vi "Destroy Broadcast Events.vi"(8 "error in (no error)":errorcluster) -> (0 "error out":errorcluster)   [LabVIEW 2015, in "Thermal Chamber Controller_DQMH.lvlib"]
doc: "Destroy the broadcast events, even if there is an incoming error.\n\n<b>NOTE</b>: The contents of this VI are automatically generated and modified by the <b>Tools > Delacor > DQMH</b> utilities. Consider using those utilities instead of making your own modifications to this VI.\n_____\nBased on Delacor QMH Project Template 2.0.0.62.\n____\nDelacor QMH Thermal Chamber Examples 4.0.0.21\nCopyright (c) 2018, Delacor"
uses:
  Thermal Chamber Controller_DQMH.lvlib
panel:
  # "NOTE: The contents of this VI are automatically generated and modified by the Tools > Delacor > DQMH utilities. Consider using those utilities instead of making your own modifications to this VI."
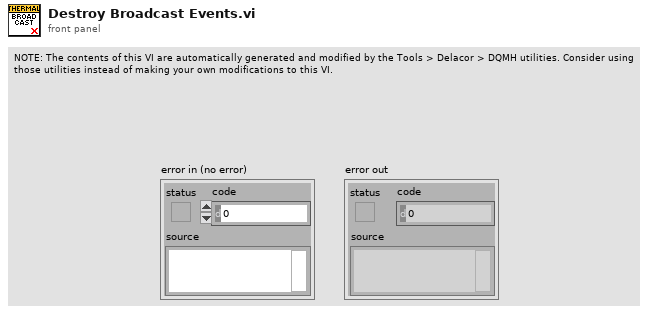
[diagram p1: front panel]
types:
  T1 = typedef "Thermal Chamber Controller_DQMH.lvlib/Broadcast Events--cluster.ctl" = cluster{"Module Did Init":refnum<user-event>, "Status Updated":refnum<user-event>, "Error Reported":refnum<user-event>, "Module Did Stop":refnum<user-event>, "Update Module Execution Status":refnum<user-event>, "Set Point Updated":refnum<user-event>, "Ramp Rate Updated":refnum<user-event>, "Heater State Updated":refnum<user-event>, "Chamber Status Updated":refnum<user-event>}
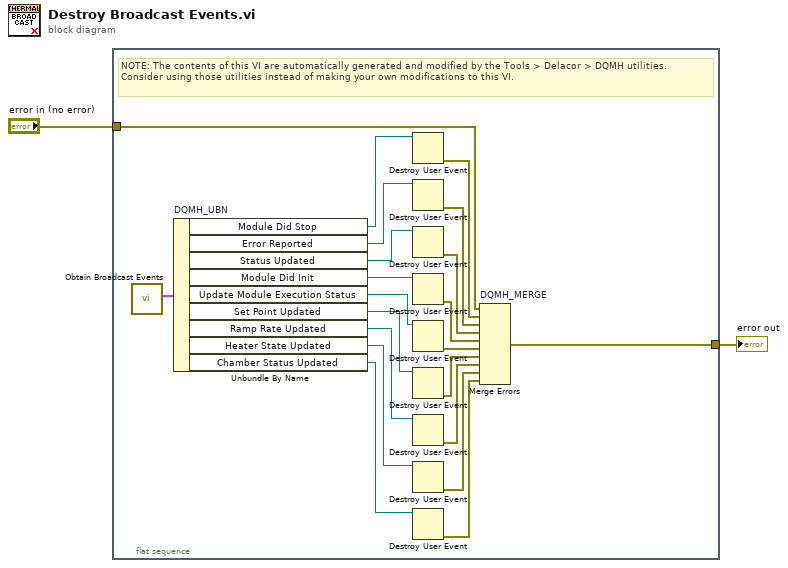
[diagram p0: block diagram]
diagram:
  n1 = flat-sequence {
    tunnel: [w22] -> w2
    tunnel: "error in (no error)" -> [w13]
    frame #0 {
      # "NOTE: The contents of this VI are automatically generated and modified by the Tools > Delacor > DQMH utilities. Consider using those utilities instead of making your own modifications to this VI."
      n2 = call "Obtain Broadcast Events.vi"() -> ("Thermal Chamber Controller_DQMH Broadcast Events"=w21:T1)  [unwired: 10 in, 1 out]
      n3 = Unbundle By Name "DQMH_UBN"(w21) -> ("Module Did Stop"=w14:refnum<user-event>, "Error Reported"=w16:refnum<user-event>, "Status Updated"=w19:refnum<user-event>, "Module Did Init"=w20:refnum<user-event>, "Update Module Execution Status"=w11:refnum<user-event>, "Set Point Updated"=w9:refnum<user-event>, "Ramp Rate Updated"=w7:refnum<user-event>, "Heater State Updated"=w5:refnum<user-event>, "Chamber Status Updated"=w3:refnum<user-event>)
      n4 = Destroy User Event(user event=w14) -> (error out=w15:errorcluster)  [unwired: 1 in]
      n5 = Destroy User Event(user event=w16) -> (error out=w17:errorcluster)  [unwired: 1 in]
      n6 = Destroy User Event(user event=w19) -> (error out=w18:errorcluster)  [unwired: 1 in]
      n7 = Destroy User Event(user event=w20) -> (error out=w23:errorcluster)  [unwired: 1 in]
      n8 = Destroy User Event(user event=w11) -> (error out=w12:errorcluster)  [unwired: 1 in]
      n9 = Destroy User Event(user event=w9) -> (error out=w10:errorcluster)  [unwired: 1 in]
      n10 = Destroy User Event(user event=w7) -> (error out=w8:errorcluster)  [unwired: 1 in]
      n11 = Destroy User Event(user event=w5) -> (error out=w6:errorcluster)  [unwired: 1 in]
      n12 = Destroy User Event(user event=w3) -> (error out=w4:errorcluster)  [unwired: 1 in]
      n13 = Merge Errors "DQMH_MERGE"(w13, w15, w17, w18, w23, w12, w10, w8, w6, w4) -> (w22:errorcluster)
    }
  }
  "error out" <- w2
